vi "Update Data Rate Divisor.vi"(8 "error in":errorcluster, 10 "Rate":dbl, 11 "objects":T1) -> (0 "error out":errorcluster)   [LabVIEW 2014]
uses:
  <vilib>/NI/DCAF/Tag Editor Core/Table API/Table Manager/object ref.ctl
  <vilib>/NI/DCAF/Tag Editor Core/Configuration Editor/Classes/Engine Parent/Engine Parent Editor Node.lvclass
  <vilib>/NI/DCAF/Tag Editor Core/Configuration Editor/Classes/Module editor node/module editor node.lvclass
  module/configuration/Write Data Rate.vi
  DAQmx Module Editor Node.lvclass
  module/configuration/DAQmx Module Configuration.lvclass
  <vilib>/NI/DCAF/Tag Editor Core/Table API/Table Manager/Table Manager.lvclass
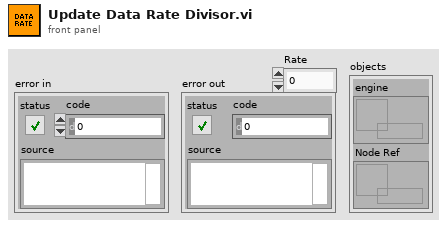
[diagram p1: front panel]
types:
  T1 = typedef "Table Manager.lvlib/Table Manager.lvclass/object ref.ctl" = cluster{"engine":refnum<data-value>, "Node Ref":refnum<data-value>}
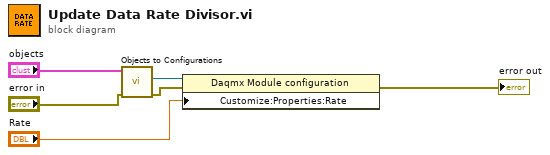
[diagram p0: block diagram]
diagram:
  n1 = call "Objects to Configurations.vi"("error in (no error)"="error in", "Objects in"="objects") -> ("error out"=w3:errorcluster, "tag bus configurable plugin module configuration"=w6:refnum<class "DAQmx Module Configuration.lvclass">)  [unwired: 7 in, 1 out]
  n2 = property class="Daqmx Module configuration"(reference=w6, error in=w3, "Customize:Properties:Rate"="Rate") -> (error out=→"error out":errorcluster)  [unwired: 1 out]
